vi "Coordinates_to_Heading_SubVI.vi"(0 "Destination (degrees)":cluster{"Latitude":dbl, "Longitude":dbl}, 2 "Current Location (degrees)":cluster{"Latitude":dbl, "Longitude":dbl}) -> (1 "Bearing":dbl, 3 "Distance":dbl)   [LabVIEW 2015]
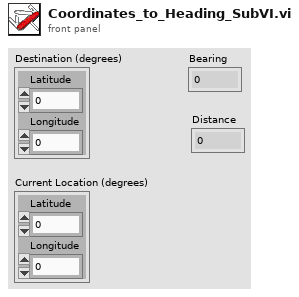
[diagram p1: front panel]
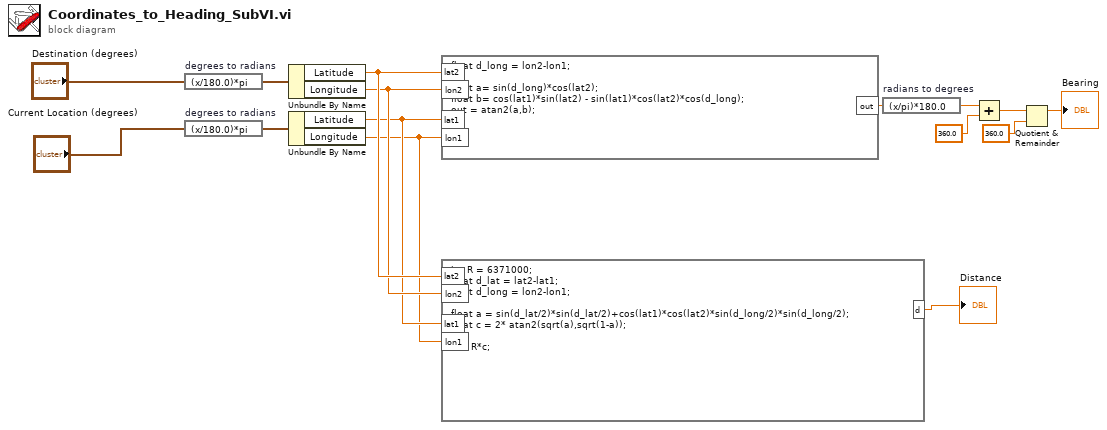
[diagram p0: block diagram]
diagram:
  n1 = expression code="(x/180.0)*pi" "degrees to radians"("Destination (degrees)") -> (w6:cluster{"Latitude":dbl, "Longitude":dbl})
  n2 = expression code="(x/180.0)*pi" "degrees to radians"("Current Location (degrees)") -> (w7:cluster{"Latitude":dbl, "Longitude":dbl})
  n3 = Unbundle By Name(w6) -> ("Latitude"=w5:dbl, "Longitude"=w4:dbl)
  n4 = Unbundle By Name(w7) -> ("Latitude"=w3:dbl, "Longitude"=w2:dbl)
  n5 = formula code="float d_long = lon2-lon1;\n\nfloat a= sin(d_long)*cos(lat2);\nfloat b= cos(lat1)*sin(lat2) - sin(lat1)*cos(lat2)*cos(d_long);\nout = atan2(a,b);"("lat1"=w3, "lat2"=w5, "lon1"=w2, "lon2"=w4) -> ("out"=w8:dbl)
  n6 = formula code="int R = 6371000;\nfloat d_lat = lat2-lat1;\nfloat d_long = lon2-lon1;\n\nfloat a = sin(d_lat/2)*sin(d_lat/2)+cos(lat1)*cos(lat2)*sin(d_long/2)*sin(d_long/2);\nfloat c = 2* atan2(sqrt(a),sqrt(1-a));\n\nd = R*c;"("lat1"=w3, "lat2"=w5, "lon1"=w2, "lon2"=w4) -> ("d"=→"Distance":dbl)
  n7 = expression code="(x/pi)*180.0" "radians to degrees"(w8) -> (w13:dbl)
  n8 = Add(x=w13, y=360.0) -> (x+y=w10:dbl)
  n9 = Quotient & Remainder(x=w10, y=360.0) -> (x-y*floor(x/y)=→"Bearing":dbl)  [unwired: 1 out]
